vi "Read Items ref.vi"(8 "error in (no error)":errorcluster, 11 "Sequence Element in":refnum<class "Sequence Element.lvclass">) -> (0 "error out":errorcluster, 2 "Items ref":refnum<vi>, 3 "Sequence Element out":refnum<class "Sequence Element.lvclass">)   [LabVIEW 2019, in "Sequence Element.lvclass"]
uses:
  Sequence Element.lvclass
  Sequence Element.lvclass/Sequence Element.ctl
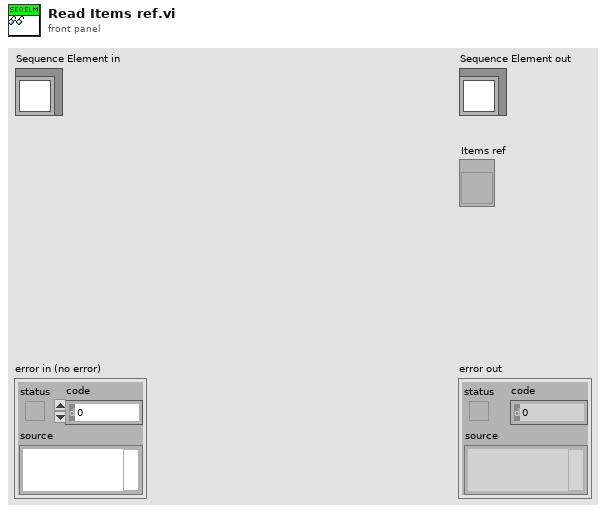
[diagram p1: front panel]
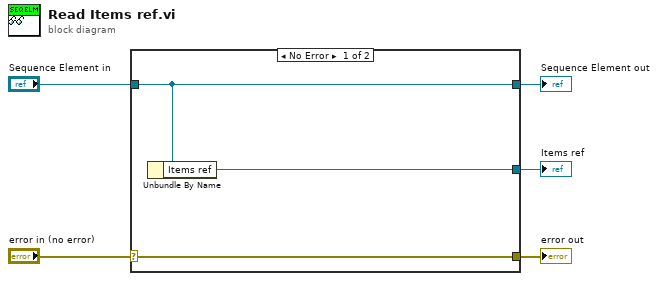
[diagram p0: block diagram]
diagram:
  n1 = case shown="No Error" "error in (no error)" {
    selector: "error in (no error)" -> [w8 w9]
    tunnel: [w8 w9] -> w4
    tunnel: [w7 w10] -> w2
    tunnel: "Sequence Element in" -> [w7 w10]
    tunnel: [w6 _] -> w1
    frame No Error {
      n2 = Unbundle By Name(w7) -> ("Items ref"=w6:refnum<vi>)
    }
    frame Error {
    }
  }
  "error out" <- w4
  "Sequence Element out" <- w2
  "Items ref" <- w1
